vi "RSZVB Set Calibration Kit With Label.vi"(7 "Calibration Kit Label (\"\")":string, 8 "error in (no error)":errorcluster {"code" format="%.0x"}, 9 "Calibration Kit Name (\"\")":string, 10 "Connector (N 50 Ohm)":i32(ring) items=["N 50 Ohm", "N 75 Ohm", "PC 7", "PC 3.5", "2.92 mm", "User 1", "User 2", "SMA"], 11 "VISA session":refnum<visa-resource-name>) -> (0 "error out":errorcluster {"code" format="%.0x"}, 3 "dup VISA session":refnum<visa-resource-name>)   [LabVIEW 2011]
doc: "This VI selects the calibration kit to be used for a specified connector type. The kit is identified by its name and label. \n\nRemote-control command(s):\n[SENSe<Ch>:]CORRection:CKIT:<conn_type>:LSELect '<ckit_name>', '<ckit_label>'"
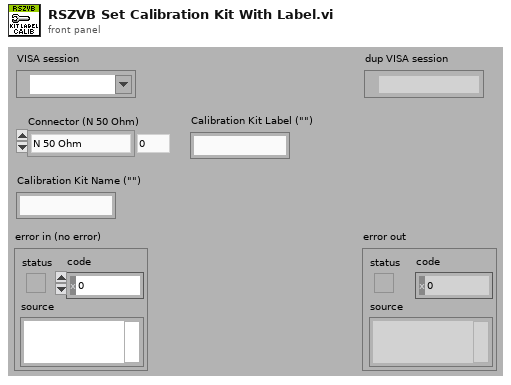
[diagram p1: front panel]
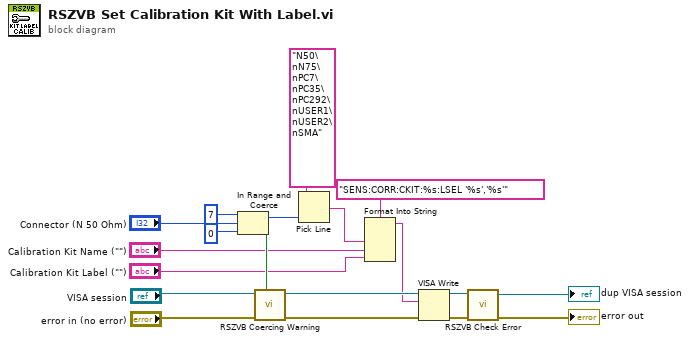
[diagram p0: block diagram]
diagram:
  n1 = In Range and Coerce(upper limit=7 ("lower limit"), x="Connector (N 50 Ohm)", lower limit=0) -> (coerced(x)=w11:i32, In Range?=w14:bool)
  n2 = call "RSZVB Coercing Warning.vi"("In Range?"=w14, "error in (no error)"="error in (no error)", "VISA session"="VISA session") -> ("error out"=w18:errorcluster, "dup VISA session"=w19:refnum<visa-resource-name>)  [unwired: 7 in]
  n3 = Pick Line(multi-line string="N50\nN75\nPC7\nPC35\nPC292\nUSER1\nUSER2\nSMA", line index=w11) -> (output string=w9:string)  [unwired: 1 in]
  n4 = Format Into String(format string="SENS:CORR:CKIT:%s:LSEL '%s','%s'", w9, "Calibration Kit Name (\"\")", "Calibration Kit Label (\"\")") -> (resulting string=w8:string)  [unwired: 2 in, 1 out]
  n5 = VISA Write(VISA resource name=w19, write buffer=w8, error in (no error)=w18) -> (VISA resource name out=w16:refnum<visa-resource-name>, error out=w17:errorcluster)  [unwired: 1 out]
  n6 = call "RSZVB Check Error.vi"("error in (no error)"=w17, "VISA session"=w16) -> ("error out"=→"error out":errorcluster, "dup VISA session"=→"dup VISA session":refnum<visa-resource-name>)  [unwired: 8 in]
